vi "Read.vi"(8 "error in (no error)":errorcluster, 11 "MicroDAQ.lvlib:Encoder.lvclass":refnum<class "Encoder.lvclass">) -> (0 "error out":errorcluster, 1 "position":i32, 2 "direction":enum16{"None", "CW", "CCW"}(ring), 3 "MicroDAQ.lvlib:Encoder.lvclass out":refnum<class "Encoder.lvclass">)   [LabVIEW 2009, in "MicroDAQ.lvlib" / "Encoder.lvclass"]
uses:
  <instrlib>/MicroDAQ/Channel/Encoder/Encoder.lvclass
  <instrlib>/MicroDAQ/Channel/Encoder/Create.vi
  <instrlib>/MicroDAQ/Channel/Encoder/Encoder.lvclass/Encoder.ctl
  <instrlib>/MicroDAQ/Mlink library wraper/mlink.lvlib
  <instrlib>/MicroDAQ/Channel/Channel.lvclass
  <instrlib>/MicroDAQ/MicroDAQ.lvlib
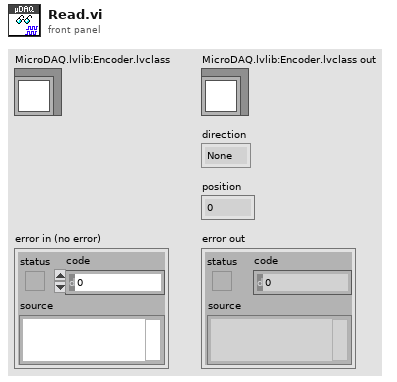
[diagram p1: front panel]
types:
  T1 = typedef "MicroDAQ.lvlib/Encoder type.ctl" = u8
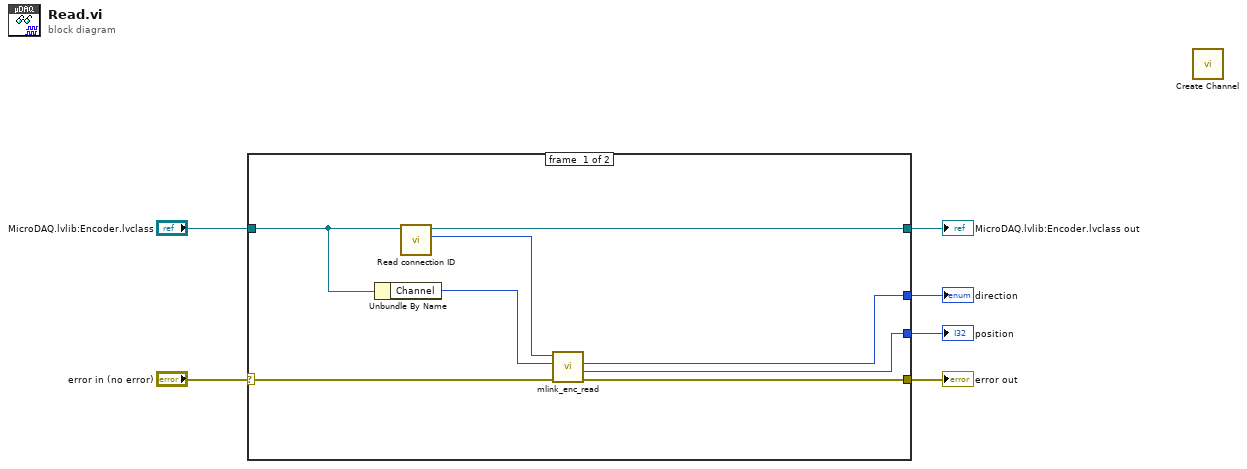
[diagram p0: block diagram]
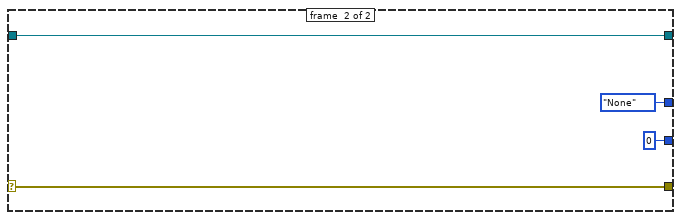
[diagram p2: hidden frame]
diagram:
  n1 = case shown="No Error" "error in (no error)" {
    selector: "error in (no error)" -> [w14 w18]
    tunnel: [w13 w18] -> w5
    tunnel: "MicroDAQ.lvlib:Encoder.lvclass" -> [w10 w17]
    tunnel: [w12 w17] -> w3
    tunnel: [w8 0 ("position")] -> w2
    tunnel: [w7 enum16{"None", "CW", "CCW"}."None" ("direction")] -> w1
    frame #0 {
      n2 = Unbundle By Name(w10) -> ("Channel"=w9:T1)
      n3 = call <instrlib>:"Read connection ID.vi"("Task in"=w10) -> ("connection ID"=w11:i32, "Task out"=w12:refnum<class "Encoder.lvclass">)  [unwired: 9 in]
      n4 = call <instrlib>:"mlink_enc_read.vi"("error in (no error)"=w14, "channel"=w9, "connection ID"=w11) -> ("error out"=w13:errorcluster, "position"=w8:i32, "direction"=w7:enum16{"None", "CW", "CCW"})  [unwired: 5 in, 1 out]
    }
    frame #1 {
    }
  }
  "MicroDAQ.lvlib:Encoder.lvclass out" <- w3
  "error out" <- w5
  "direction" <- w1
  "position" <- w2
  n5 = call-poly <instrlib>:"Create Channel.vi"() -> ()  [unwired: 10 in, 2 out]
